vi "Actor Core.vi"(8 "error in":errorcluster, 11 "Launch IMAQ Display in":refnum<class "Camera Display.lvclass">) -> (0 "error out":errorcluster, 3 "Actor out":refnum<class "Actor.lvclass">)   [LabVIEW 2014, in "Camera Display.lvlib" / "Camera Display.lvclass"]
doc: "(<B>Filename</B>: Actor Framework.lvlib:Actor.lvclass:Actor Core.vi)\n\nReceives messages to the actor, reacts to them, and initiates any error handling that may shut the actor down.\n\nDescendant classes may override this VI to append parallel tasks for the actor to complete while it handles messages. Overrides use the Call Parent Method node."
uses:
  Camera Display.lvclass
  <vilib>/ActorFramework/Actor/Actor.lvclass
  <vilib>/userdefined/High Color/IMAQdx.ctl
  Analyze Classes/Analyze Diviation/Analyze BeamDeviation.lvclass
  IMAQdx Actor/IMAQdx Actor/IMAQdx Actor.lvclass
  HIJ Vision Display/HIJ Vision Display Messages/New Image Msg/New Image Msg.lvclass
  HIJ IMAQdx Display/AF IMAQ Display/HIJ IMAQdx Display.lvclass
  Camera Display.lvclass/Camera Display.ctl
  HIJ Vision Display/HIJ Vision Display/HIJ Vision Display.lvclass/HIJ Vision Display.ctl
  HIJ IMAQdx Display/AF IMAQ Display/HIJ IMAQdx Display.lvclass/HIJ IMAQdx Display.ctl
  Camera Actor/Camera Actor Messages/Start Acquisition Msg/Start Acquisition Msg.lvclass/Start Acquisition Msg.ctl
  <vilib>/ActorFramework/Message Enqueuer/Message Enqueuer.lvclass/Message Enqueuer.ctl
  <vilib>/ActorFramework/Actor/Actor.lvclass/Actor.ctl
  Camera Actor/Camera Actor Messages/Write Receiver Params Msg/Write Receiver Params Msg.lvclass/Write Receiver Params Msg.ctl
  Shared Code/Viewable Actor/ViewableActor Messages/Insert Into SubPanel Msg/Insert Into SubPanel Msg.lvclass/Insert Into SubPanel Msg.ctl
  Camera Actor/Camera Actor Messages/Change Camera Msg/Change Camera Msg.lvclass/Change Camera Msg.ctl
  HIJ Vision Display/HIJ Vision Display Messages/Change Image Source Msg/Change Image Source Msg.lvclass/Change Image Source Msg.ctl
  HIJ Vision Display/HIJ Vision Display Messages/Write Image Name Prefix Msg/Write Image Name Prefix Msg.lvclass/Write Image Name Prefix Msg.ctl
  HIJ Vision Display/HIJ Vision Display/Write Image Source Name.vi
  HIJ IMAQdx Display/AF IMAQ Display/Write ConfigDir.vi
  HIJ Vision Display/HIJ Vision Display/Write Save Report_.vi
  HIJ Vision Display/HIJ Vision Display/Write Show ZoomBtn_.vi
  HIJ Vision Display/HIJ Vision Display/Write WorkDir.vi
  <vilib>/ActorFramework/Message Enqueuer/Enqueue.vi
  <vilib>/ActorFramework/Message Enqueuer/Init from Existing Queue.vi
  <vilib>/ActorFramework/Message Priority Queue/Priority Enqueue.vi
  Camera Actor/Camera Actor Messages/Start Acquisition Msg/Start Acquisition Msg.lvclass
  <vilib>/ActorFramework/Message Enqueuer/Message Enqueuer.lvclass
  Camera Actor/Camera Actor Messages/Write Receiver Params Msg/Write Receiver Params Msg.lvclass
  Shared Code/Viewable Actor/ViewableActor Messages/Insert Into SubPanel Msg/Insert Into SubPanel Msg.lvclass
  Camera Actor/Camera Actor Messages/Stop Acquisition Msg/Stop Acquisition Msg.lvclass
  Camera Actor/Camera Actor Messages/Change Camera Msg/Change Camera Msg.lvclass
  HIJ Vision Display/HIJ Vision Display Messages/Change Image Source Msg/Change Image Source Msg.lvclass
  <vilib>/ActorFramework/Stop Msg/Stop Msg.lvclass
  HIJ Vision Display/HIJ Vision Display Messages/Write Image Name Prefix Msg/Write Image Name Prefix Msg.lvclass
  HIJ Vision Display/HIJ Vision Display Messages/Save Image Msg/Save Image Msg.lvclass
  Shared Code/Viewable Actor/ViewableActor/ViewableActor.lvclass
panel:
  in  "Settings":bool
  in  "Camera":T1
  in  "Stop Button":bool
  in  "Save":bool
  in  "Prefix":string
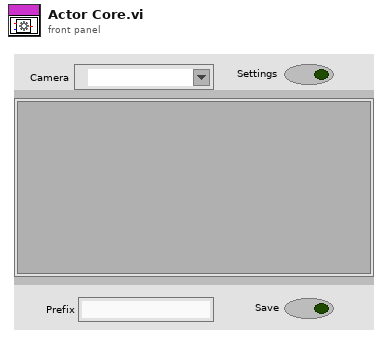
[diagram p1: front panel]
types:
  T1 = typedef "IMAQdx.ctl" = refnum<k21>
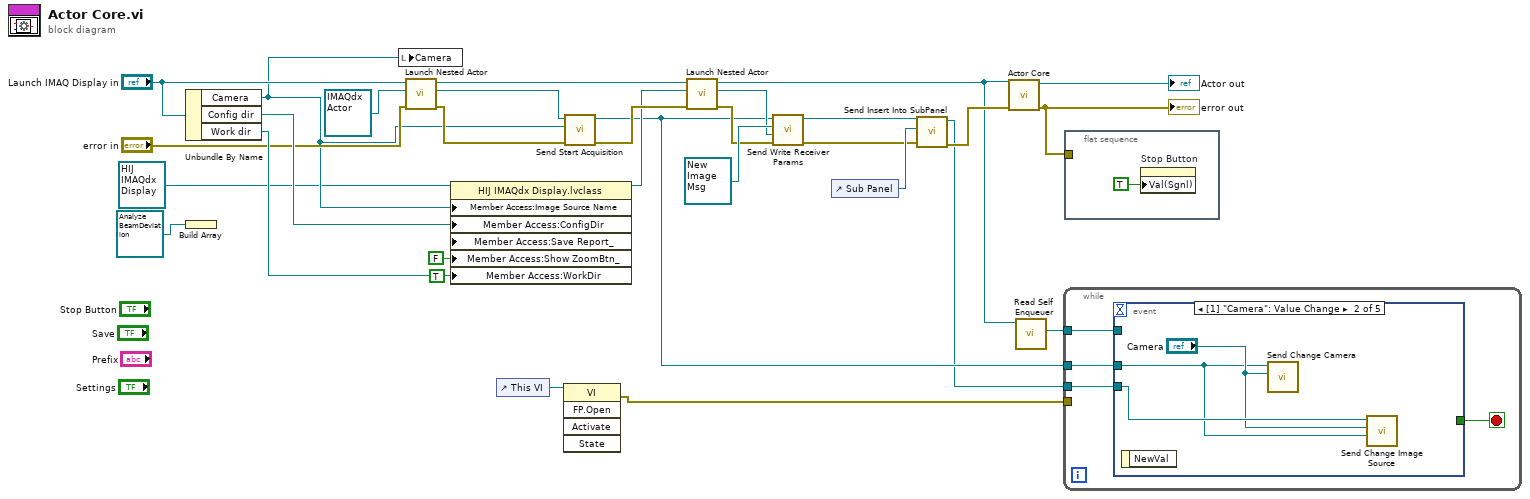
[diagram p0: block diagram]
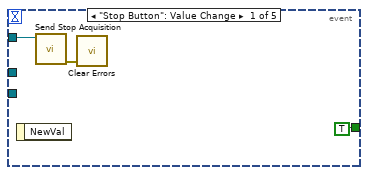
[diagram p2: hidden frame]
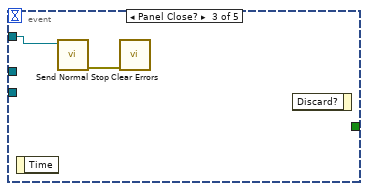
[diagram p3: hidden frame]
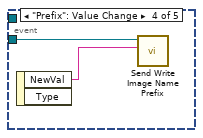
[diagram p4: hidden frame]
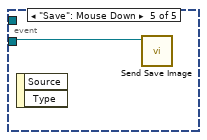
[diagram p5: hidden frame]
diagram:
  n1 = Unbundle By Name("Launch IMAQ Display in") -> ("Camera"=w3:T1, "Config dir"=w30:path, "Work dir"=w29:path)
  n2 = Build Array(refnum<class "Analyze BeamDeviation.lvclass"> refnum ("Analyze.lvlib:Analyze BeamDeviation.lvclass")) -> ()  [unwired: 1 out]
  n3 = local write "Camera"(w3) -> ()
  n4 = call <vilib>:"Launch Nested Actor.vi"("error in (no error)"="error in", "Nested Actor"=refnum<class "IMAQdx Actor.lvclass"> refnum ("IMAQdx Actor.lvlib:IMAQdx Actor.lvclass"), "Caller Actor in"="Launch IMAQ Display in") -> ("error out"=w19:errorcluster, "Nested Actor's Enqueuer"=w18:refnum<class "Message Enqueuer.lvclass">, "Caller Actor out"=w13:refnum<class "Camera Display.lvclass">)  [unwired: 6 in]
  n5 = property class="HIJ IMAQdx Display.lvclass"(reference=refnum<class "HIJ IMAQdx Display.lvclass"> refnum ("HIJ IMAQdx Display.lvlib:HIJ IMAQdx Display.lvclass"), "Member Access:Image Source Name"=w3, "Member Access:ConfigDir"=w30, "Member Access:Save Report_"=FALSE ("Save Report_"), "Member Access:Show ZoomBtn_"=TRUE ("Show ZoomBtn_"), "Member Access:WorkDir"=w29) -> (reference out=w9:refnum<class "HIJ IMAQdx Display.lvclass">)  [unwired: 1 in, 1 out]
  n6 = control-ref of="This VI"() -> (w20:refnum<vi>)
  n7 = invoke class="VI" method="FP.Open"(reference=w20) -> (error out=w2:errorcluster)  [unwired: 4 in, 4 out]
  n8 = call "Send Start Acquisition.vi"("error in (no error)"=w19, "Camera Name"=w3, "Message Enqueuer"=w18) -> ("error out"=w11:errorcluster, "Message Enqueuer out"=w6:refnum<class "Message Enqueuer.lvclass">)  [unwired: 7 in]
  n9 = call <vilib>:"Launch Nested Actor.vi"("error in (no error)"=w11, "Nested Actor"=w9, "Caller Actor in"=w13) -> ("error out"=w10:errorcluster, "Nested Actor's Enqueuer"=w8:refnum<class "Message Enqueuer.lvclass">, "Caller Actor out"=w12:refnum<class "Camera Display.lvclass">)  [unwired: 6 in]
  n10 = call "Send Write Receiver Params.vi"("error in (no error)"=w10, "Image Receiver"=w8, "New Image Msg"=refnum<class "New Image Msg.lvclass"> refnum ("AF IMAQ Display.lvlib:New Image Msg.lvclass"), "Message Enqueuer"=w6) -> ("error out"=w15:errorcluster, "Message Enqueuer out"=w7:refnum<class "Message Enqueuer.lvclass">)  [unwired: 6 in]
  n11 = control-ref of="Sub Panel"() -> (w27:refnum<vi>)
  n12 = call "Send Insert Into SubPanel.vi"("error in (no error)"=w15, "SubPanel Ref"=w27, "Message Enqueuer"=w7) -> ("error out"=w26:errorcluster, "Message Enqueuer out"=w5:refnum<class "Message Enqueuer.lvclass">)  [unwired: 7 in]
  n13 = call-parent "Actor Core.vi"("error in"=w26, "Actor in"=w12) -> ("error out"=w25:errorcluster, "Actor out"=→"Actor out":refnum<class "Actor.lvclass">)  [unwired: 8 in]
  "error out" <- w25
  n14 = call <vilib>:"Read Self Enqueuer.vi"("Actor"=w12) -> ("Self Enqueuer"=w24:refnum<class "Message Enqueuer.lvclass">)  [unwired: 10 in]
  n15 = while {
    tunnel: w24 -> [w33]
    tunnel: w6 -> [w32]
    tunnel: w5 -> [w31]
    tunnel: w2 -> [_]
    stop <- w34 stop-if-true
    n16 = event shown="[1] \"Camera\": Value Change" {
      selector: _ -> [_ _ _ _ _]
      dyn-events: _ -> [_ _ _ _ _]
      timeout: _ -> [_ _ _ _ _]
      tunnel: [TRUE _ _ _ _] -> w34
      tunnel: w33 -> [w36 _ w41 _ _]
      tunnel: w32 -> [_ w38 _ _ _]
      tunnel: w31 -> [_ w40 _ w44 w45]
      event "Stop Button": Value Change {
        n17 = event-data() -> ()  [unwired: 1 in, 1 out]
        n18 = call "Send Stop Acquisition.vi"("Message Enqueuer"=w36) -> ("error out"=w35:errorcluster)  [unwired: 9 in, 1 out]
        n19 = call <vilib>:"Clear Errors.vi"("error in (no error)"=w35) -> ()  [unwired: 5 in, 2 out]
      }
      event Value Change {
        n20 = event-data() -> ()  [unwired: 1 in, 1 out]
        n21 = call "Send Change Camera.vi"("New Camera"="Camera", "Message Enqueuer"=w38) -> ()  [unwired: 8 in, 2 out]
        n22 = call "Send Change Image Source.vi"("Image Source Enq"=w38, "Image Source"="Camera", "Message Enqueuer"=w40) -> ()  [unwired: 7 in, 2 out]
      }
      event Panel Close? {
        n23 = event-data() -> ()  [unwired: 1 in, 1 out]
        n24 = call <vilib>:"Send Normal Stop.vi"("Message Enqueuer"=w41) -> ("error out"=w42:errorcluster)  [unwired: 10 in]
        n25 = call <vilib>:"Clear Errors.vi"("error in (no error)"=w42) -> ()  [unwired: 5 in, 2 out]
        n26 = event-data() -> ()  [unwired: 2 in, 1 out]
      }
      event "Prefix": Value Change {
        n27 = event-data() -> ("NewVal"=w43:string)  [unwired: 1 in, 1 out]
        n28 = call "Send Write Image Name Prefix.vi"("Image Name Prefix"=w43, "Message Enqueuer"=w44) -> ()  [unwired: 8 in, 2 out]
      }
      event "Save": Mouse Down {
        n29 = event-data() -> ()  [unwired: 1 in, 2 out]
        n30 = call "Send Save Image.vi"("Message Enqueuer"=w45) -> ()  [unwired: 9 in, 2 out]
      }
    }
  }
  n31 = flat-sequence {
    tunnel: w25 -> [_]
    frame #0 {
      n32 = property on="Stop Button" class="Bool (strict)"("Val(Sgnl)"=TRUE) -> ()  [unwired: 2 in, 2 out]
    }
  }
